vi "MdfSetChannelValue.vi"(6 "currentTime":u64, 7 "deltT":u64=10, 8 "error in (no error)":errorcluster, 9 "setValues":dbl[](array[numeric]), 10 "ChannelGroupRef in":refnum<k24>, 11 "MDFRef":refnum<k24>) -> (0 "error out":errorcluster, 2 "endTime":u64, 3 "MDFRef out":refnum<k24>)   [LabVIEW 2025, in "MdfFile.lvlib"]
uses:
  MdfFile.lvlib
  data/mdflibrary.dll
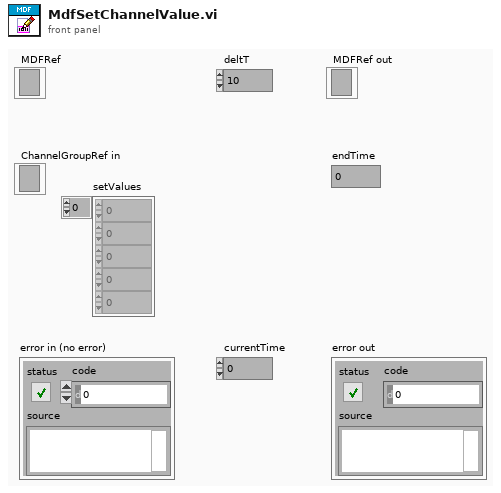
[diagram p1: front panel]
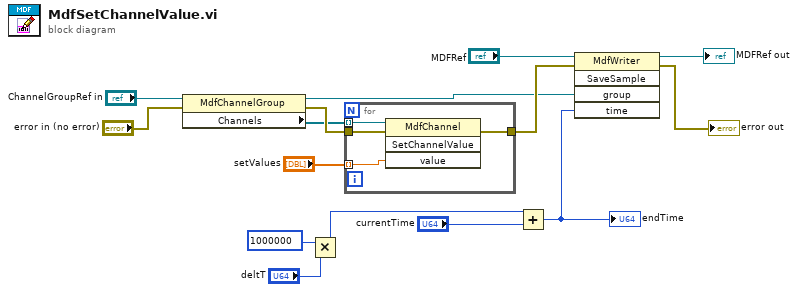
[diagram p0: block diagram]
diagram:
  n1 = property class="MdfChannelGroup"(reference="ChannelGroupRef in", error in="error in (no error)") -> (reference out=w5:refnum<k24>, error out=w15:errorcluster, "Channels"=w12:refnum<k24>[])
  n2 = Multiply(x=u64 1000000 ("y"), y="deltT") -> (x*y=w1:u64)
  n3 = for {
    tunnel: w12 -> [w18] mode=indexing
    tunnel: "setValues" -> [w17] mode=indexing
    tunnel: w15 -> [w19]
    tunnel: [w16] -> w7
    n4 = invoke class="MdfChannel" method="SetChannelValue"(reference=w18, error in=w19, "value"=w17) -> (error out=w16:errorcluster)  [unwired: 1 in, 3 out]
  }
  n5 = Add(x=w1, y="currentTime") -> (x+y=w4:u64)
  "endTime" <- w4
  n6 = invoke class="MdfWriter" method="SaveSample"(reference="MDFRef", error in=w7, "group"=w5, "time"=w4) -> (reference out=→"MDFRef out":refnum<k24>, error out=→"error out":errorcluster)  [unwired: 1 in, 3 out]
